vi "Analog Output Write.vi"(8 "error in":errorcluster, 10 "Waveform Output Write":dbl[](array[numeric]) format="%0.2f", 11 "NI Waveform Output in":refnum<class "NI Waveform Output.lvclass">) -> (0 "error out":errorcluster, 3 "NI Waveform Output out":refnum<class "NI Waveform Output.lvclass">)   [LabVIEW 2023, in "HardwareAbstractionLayer_LVOOP.lvlib" / "NI Waveform Output.lvclass"]
uses:
  NI Waveform Output.lvclass
  NI Waveform Output.lvclass/NI Waveform Output.ctl
  <vilib>/DAQmx/write.llb/DAQmx Write (Analog 1D DBL NChan 1Samp).vi
  <vilib>/DAQmx/miscellaneous.llb/DAQmx Fill In Error Info.vi
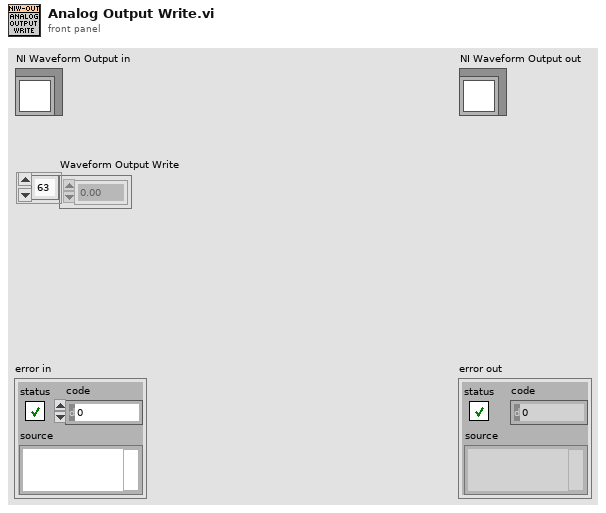
[diagram p1: front panel]
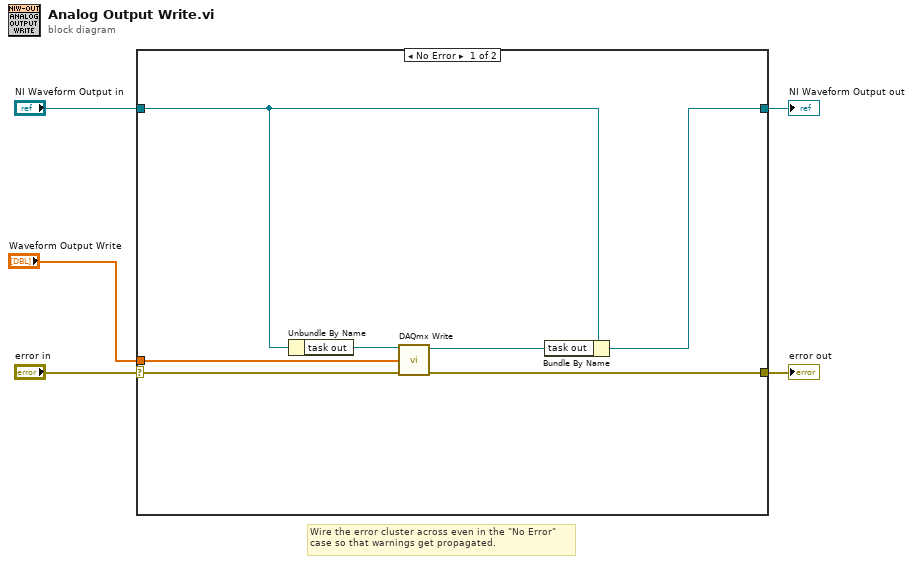
[diagram p0: block diagram]
diagram:
  # "Wire the error cluster across even in the \"No Error\"\ncase so that warnings get propagated."
  n1 = case shown="No Error" "error in" {
    selector: "error in" -> [w12 w14]
    tunnel: [w11 w14] -> w4
    tunnel: [w8 w13] -> w2
    tunnel: "NI Waveform Output in" -> [w9 w13]
    tunnel: "Waveform Output Write" -> [w10 _]
    frame No Error {
      n2 = Unbundle By Name(w9) -> ("task out"=w6:refnum<k21>)
      n3 = call-poly <vilib>:"DAQmx Write.vi"("task/channels in"=w6, "data"=w10, "error in"=w12) -> ("task out"=w7:refnum<k21>, "error out"=w11:errorcluster)  [unwired: 10 in, 1 out]
      n4 = Bundle By Name(cluster=w9, "task out"=w7) -> (w8:refnum<class "NI Waveform Output.lvclass">)
    }
    frame Error {
    }
  }
  "error out" <- w4
  "NI Waveform Output out" <- w2
